vi "CAN DB test.vi"() -> ()   [LabVIEW 2021]
uses:
  CAN/CAN.lvclass
panel:
  out "Current":dbl[][](array[numeric])
  out "Voltage":dbl[][](array[numeric])
  in  "stop":bool
  in  "Box IDs":u8[](array[numeric])=[1]
  in  "CAN Interface":refnum<k21>
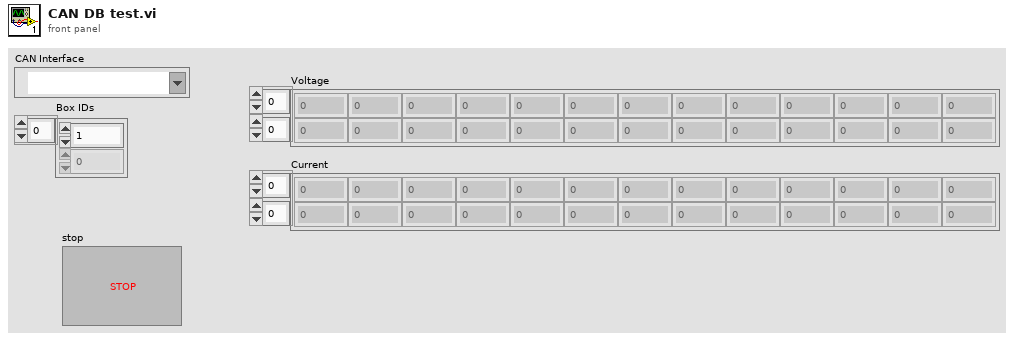
[diagram p1: front panel]
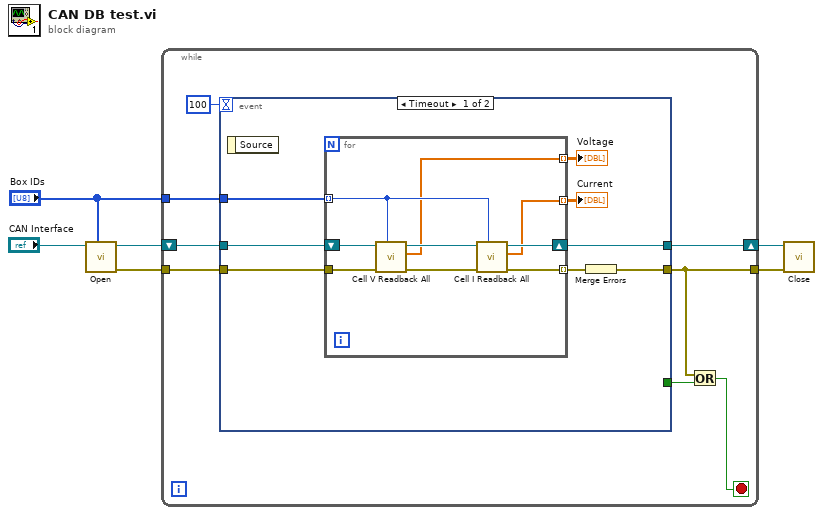
[diagram p0: block diagram]
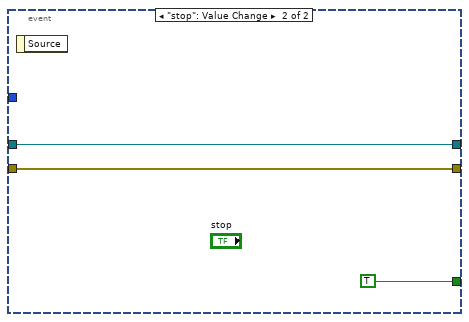
[diagram p2: hidden frame]
diagram:
  n1 = call "Open.vi"("Box IDs"="Box IDs", "CAN Interface"="CAN Interface") -> ("error out"=w4:errorcluster, "CAN out"=w3:refnum<class "CAN.lvclass">)  [unwired: 8 in]
  n2 = while {
    tunnel: "Box IDs" -> [w14]
    shift-right: [w11] -> w2
    shift-left: w3 -> [w12]
    tunnel: w4 -> [w13]
    tunnel: [w8] -> w1
    stop <- w9 stop-if-true
    n3 = event shown="[0] Timeout" {
      selector: _ -> [_ _]
      dyn-events: _ -> [_ _]
      timeout: 100 -> [_ _]
      tunnel: w14 -> [w22 _]
      tunnel: w13 -> [w21 w33]
      tunnel: w12 -> [w20 w34]
      tunnel: [w19 w34] -> w11
      tunnel: [w17 w33] -> w8
      tunnel: [_ TRUE] -> w10
      event Timeout {
        n4 = event-data() -> ()  [unwired: 1 in, 1 out]
        n5 = for {
          tunnel: w22 -> [w31] mode=indexing
          tunnel: w21 -> [w30]
          shift-right: [w26] -> w19
          shift-left: w20 -> [w28]
          tunnel: [w25] -> w18 mode=indexing
          tunnel: [w24] -> w16 mode=indexing
          tunnel: [w23] -> w15 mode=indexing
          n6 = call-dynamic "Cell V Readback All.vi"("Box ID"=w31, "error in (no error)"=w30, "CAN in"=w28) -> ("error out"=w29:errorcluster, "Voltage"=w24:dbl[], "CAN out"=w27:refnum<class "CAN.lvclass">)  [unwired: 6 in]
          n7 = call-dynamic "Cell I Readback All.vi"("Box ID"=w31, "error in (no error)"=w29, "CAN in"=w27) -> ("error out"=w25:errorcluster, "Current"=w23:dbl[], "CAN out"=w26:refnum<class "CAN.lvclass">)  [unwired: 6 in]
        }
        "Voltage" <- w16
        "Current" <- w15
        n8 = Merge Errors(w18) -> (w17:errorcluster)
      }
      event "stop": Value Change {
        n9 = event-data() -> ()  [unwired: 1 in, 1 out]
      }
    }
    n10 = Or(x=w8, y=w10) -> (x .or. y?=w9:bool)
  }
  n11 = call-dynamic "Close.vi"("error in (no error)"=w1, "CAN in"=w2) -> ()  [unwired: 9 in, 1 out]
